vi "acc_gyro_enc_logger.vi"() -> ()   [LabVIEW 2013]
uses:
  acc_gyro_enc_data.ctl
  <vilib>/Analysis/_algsub.llb/Real Vector Norm.vi
  <vilib>/Instr/_visa.llb/VISA Configure Serial Port (Instr).vi
  <vilib>/Analysis/NI_AALPro.lvlib
panel:
  out "Acc Mag":dbl caption="Acceleration\nmagnitude"
  in  "counts per rev":dbl=2048.0
  out "Encoder":waveform(dbl)(graph)
  out "Rate":dbl[unit]
  in  "Baud rate":u32=57600
  out "Accelerometer":waveform(dbl)[](graph)
  out "Gyro":waveform(dbl)[](graph)
  in  "accel range (m/s2)":dbl(ring)=2.0 items=["2"=2.0, "4"=4.0, "8"=8.0, "16"=16.0]
  in  "gyro range (deg/s)":dbl(ring)=250.0 items=["250"=250.0, "500"=500.0, "1000"=1000.0, "2000"=2000.0]
  in  "Serial port":refnum<visa-resource-name>="COM3"
  in  "stop":bool
  # "g"
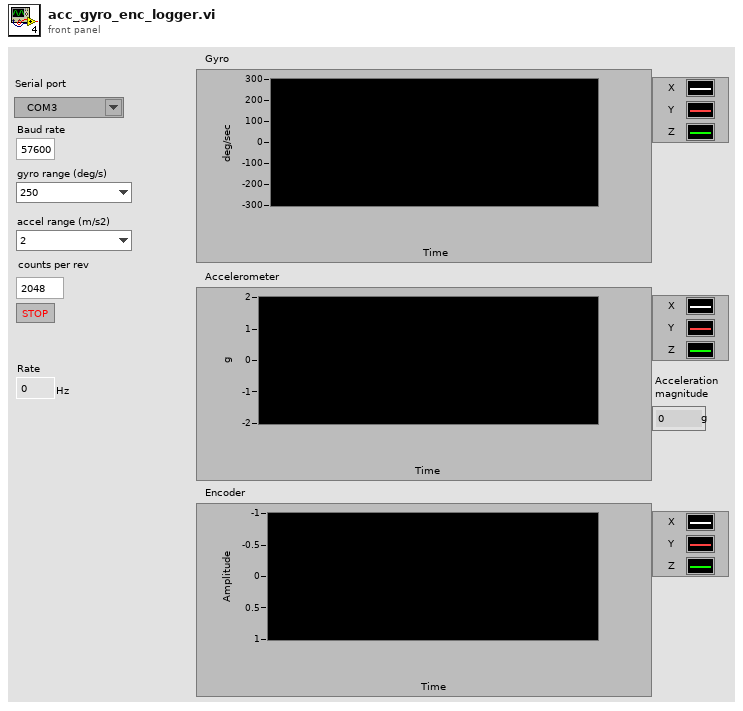
[diagram p1: front panel]
types:
  T1 = typedef "acc_gyro_enc_data.ctl" = cluster{"milliseconds":u64, "gyro_x":dbl, "gyro_y":dbl, "gyro_z":dbl, "acc_x":dbl, "acc_y":dbl, "acc_z":dbl, "encoder":dbl}
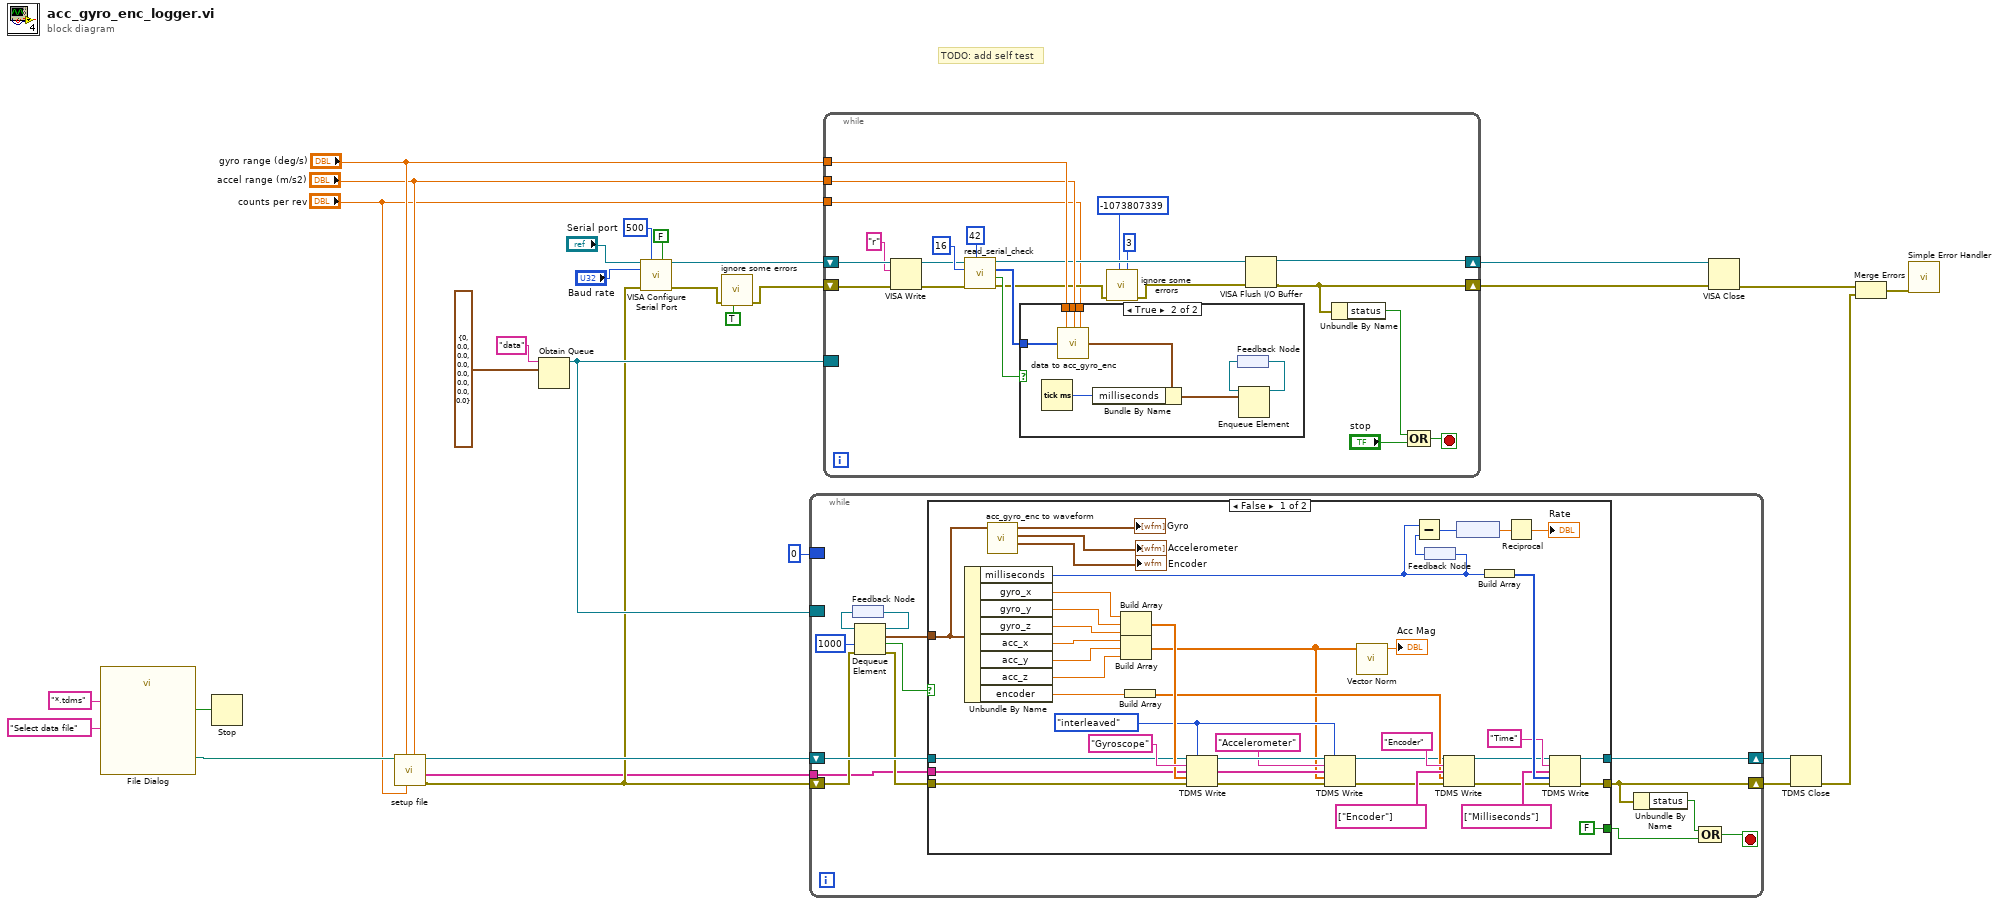
[diagram p0: block diagram]
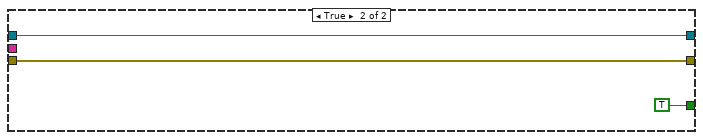
[diagram p2: hidden frame]
diagram:
  # "TODO: add self test"
  n1 = call "File Dialog"("prompt"="Select data file", "pattern (all files)"="*.tdms") -> ("selected path"=w23:path, "cancelled"=w22:bool)  [unwired: 10 in, 2 out]
  n2 = Stop(stop? (T)=w22) -> ()
  n3 = call "setup file.vi"("accel range"="accel range (m/s2)", "counts per rev"="counts per rev", "gyro range"="gyro range (deg/s)", "selected path"=w23) -> ("error out"=w12:errorcluster, "channel names"=w9:string[], "tdms file out"=w13:refnum<k34>)  [unwired: 5 in]
  n4 = Obtain Queue(name (unnamed)="data", element data type=T1 {"milliseconds"=0, "gyro_x"=0.0, "gyro_y"=0.0, "gyro_z"=0.0, "acc_x"=0.0, "acc_y"=0.0, "acc_z"=0.0, "encoder"=0.0} ("acc gyro data")) -> (queue out=w21:refnum<queue>)  [unwired: 3 in, 2 out]
  n5 = call-poly "VISA Configure Serial Port"("VISA resource name"="Serial port", "timeout (10sec)"=u32 500, "Enable Termination\nChar (T)"=FALSE ("Enable Termination\nChar (T)"), "baud rate (9600)"="Baud rate", "error in (no error)"=w12) -> ("VISA resource name out"=w6:refnum<visa-resource-name>, "error out"=w5:errorcluster)  [unwired: 9 in]
  n6 = call "ignore some errors.vi"("reset"=TRUE, "error in"=w5) -> ("error out"=w4:errorcluster)  [unwired: 8 in, 1 out]
  n7 = while {
    border: w21 -> [_]
    shift-right: [w34] -> w18
    shift-left: w12 -> [w37]
    shift-right: [w39] -> w17
    shift-left: w13 -> [w40]
    tunnel: w9 -> [w30]
    border: u64 0 ("milliseconds") -> [_]
    stop <- w31 stop-if-true
    n8 = feedback #1() -> (w43:refnum<queue>)
    n9 = Dequeue Element(queue=w43, timeout in ms (-1)=1000, error in (no error)=w37) -> (queue out=w42:refnum<queue>, element=w41:T1, timed out?=w35:bool, error out=w36:errorcluster)
    n10 = feedback-in #1(w42) -> ()
    n11 = case shown="False" w35 {
      tunnel: w41 -> [w55 _]
      tunnel: [w64 w85] -> w34
      tunnel: w40 -> [w62 w86]
      tunnel: [w63 w86] -> w39
      tunnel: w36 -> [w65 w85]
      tunnel: [FALSE TRUE] -> w32
      tunnel: w30 -> [w68 _]
      frame False {
        w61 = enum16{"decimated", "interleaved"}."interleaved" ("data layout (0:decimated)")
        n12 = Unbundle By Name(w55) -> ("milliseconds"=w60:u64, "gyro_x"=w84:dbl, "gyro_y"=w83:dbl, "gyro_z"=w82:dbl, "acc_x"=w81:dbl, "acc_y"=w80:dbl, "acc_z"=w79:dbl, "encoder"=w51:dbl)
        n13 = call "acc_gyro_enc to waveform.vi"("acc gyro data"=w55) -> ("encoder"=→"Encoder":waveform(dbl), "accel plot"=→"Accelerometer":waveform(dbl)[], "gyro plot"=→"Gyro":waveform(dbl)[])  [unwired: 8 in]
        n14 = Build Array(w84, w83, w82) -> (w71:dbl[])
        n15 = Build Array(w81, w80, w79) -> (w45:dbl[])
        n16 = Build Array(w51) -> (w50:dbl[])
        n17 = TDMS Write(0:w62, 1:w61, 5:"Gyroscope" ("group name (Untitled)"), 7:w68, 9:w71, 11:w65) -> (4:w77:refnum<k34>, 8:w67:string[], 15:w76:errorcluster)  [unwired: 1 out]
        n18 = TDMS Write(0:w77, 1:w61, 5:"Accelerometer" ("group name (Untitled)"), 7:w67, 9:w45, 11:w76) -> (4:w49:refnum<k34>, 15:w48:errorcluster)  [unwired: 2 out]
        n19 = call-poly <vilib>:"Vector Norm.vi"("Input Vector"=w45) -> ("norm"=→"Acc Mag":dbl)  [unwired: 9 in, 1 out]
        n20 = feedback #2() -> (w59:u64)
        n21 = Subtract(x=w60, y=w59) -> (x-y=w58:u64)
        n22 = feedback-in #2(w60) -> ()
        n23 = TDMS Write(0:w49, 5:"Encoder" ("group name in (Untitled)"), 7:string[] ["Encoder"] ("channel name(s) in (Untitled)"), 9:w50, 11:w48) -> (4:w47:refnum<k34>, 15:w46:errorcluster)  [unwired: 1 in, 2 out]
        n24 = node(w58) -> (w57:dbl[unit])
        n25 = Build Array(w60) -> (w74:u64[])
        n26 = Reciprocal(x=w57) -> (1/x=→"Rate":dbl[unit])
        n27 = TDMS Write(0:w47, 5:"Time" ("group name (Untitled)"), 7:string[] ["Milliseconds"] ("channel name(s) in (Untitled)"), 9:w74, 11:w46) -> (4:w63:refnum<k34>, 15:w64:errorcluster)  [unwired: 1 in, 2 out]
      }
      frame True {
      }
    }
    n28 = Unbundle By Name(w34) -> ("status"=w33:bool)
    n29 = Compound Arithmetic op=OR(w33, w32) -> (w31:bool)
  }
  n30 = while {
    tunnel: "gyro range (deg/s)" -> [w104]
    tunnel: "accel range (m/s2)" -> [w103]
    border: w21 -> [_]
    shift-right: [w93] -> w20
    shift-left: w4 -> [w100]
    shift-right: [w94] -> w19
    shift-left: w6 -> [w109]
    tunnel: "counts per rev" -> [w88]
    stop <- w97 stop-if-true
    n31 = VISA Write(VISA resource name=w109, write buffer="r", error in (no error)=w100) -> (VISA resource name out=w102:refnum<visa-resource-name>, error out=w99:errorcluster)  [unwired: 1 out]
    n32 = call "read_serial_check.vi"("checkval"=u8 42, "error in (no error)"=w99, "byte count"=u32 16, "VISA resource name"=w102) -> ("error out"=w92:errorcluster, "good"=w106:bool, "data"=w105:u8[], "VISA resource out"=w95:refnum<visa-resource-name>)  [unwired: 4 in]
    n33 = case shown="True" w106 {
      tunnel: w105 -> [_ w118]
      tunnel: w104 -> [_ w117]
      tunnel: w103 -> [_ w116]
      tunnel: w88 -> [_ w110]
      frame False {
      }
      frame True {
        n34 = Tick Count (ms)() -> (millisecond timer value=w113:u32)
        n35 = call "data to acc_gyro_enc.vi"("gyro range (deg/s)"=w117, "accel range (m/s2)"=w116, "counts per rev"=w110, "byte array"=w118) -> ("acc gyro data"=w112:T1)  [unwired: 11 in]
        n36 = Bundle By Name(cluster=w112, "milliseconds"=w113) -> (w111:T1)
        n37 = feedback #3() -> (w114:refnum<queue>)
        n38 = Enqueue Element(queue=w114, element=w111) -> (queue out=w115:refnum<queue>)  [unwired: 2 in, 2 out]
        n39 = feedback-in #3(w115) -> ()
      }
    }
    n40 = call "ignore some errors.vi"("max errors"=3, "error code"=-1073807339, "error in"=w92) -> ("error out"=w91:errorcluster)  [unwired: 7 in, 1 out]
    n41 = VISA Flush I/O Buffer(VISA resource name=w95, error in (no error)=w91) -> (VISA resource name out=w94:refnum<visa-resource-name>, error out=w93:errorcluster)  [unwired: 1 in]
    n42 = Unbundle By Name(w93) -> ("status"=w96:bool)
    n43 = Compound Arithmetic op=OR(w96, "stop") -> (w97:bool)
  }
  n44 = VISA Close(VISA resource name=w19, error in (no error)=w20) -> (error out=w16:errorcluster)
  n45 = TDMS Close(8:w18, 11:w17) -> (0:w15:errorcluster)  [unwired: 1 out]
  n46 = Merge Errors(w16, w15) -> (w14:errorcluster)
  n47 = call <vilib>:"Simple Error Handler.vi"("error in (no error)"=w14) -> ()  [unwired: 4 in, 5 out]
